vi "line_test.vi"   [LabVIEW 2012]
uses:
  <vilib>/NXT/Dual Mode Library/Display/drawLine.vi
  <vilib>/NXT/Dual Mode Library/Waits/Wait_Num.vi
types:
  T1 = cluster{"Start X":i16, "Start X":i16, "Start X":i16, "Start X":i16}
  T2 = typedef "LVHSConnector.ctl" = cluster{"Hardware":string, "Flattened String":string}
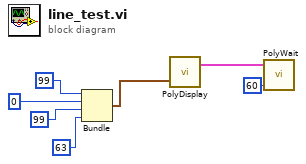
[diagram p0: block diagram]
diagram:
  n1 = Bundle("Start X"=i16 99, "Start X"=i16 0, "Start X"=i16 99, "Start X"=i16 63) -> (w4:T1)  [unwired: 1 in]
  n2 = call-poly <vilib>:"PolyDisplay.vi"("Line Parameters"=w4) -> ("NXT"=w6:T2)  [unwired: 3 in]
  n3 = call-poly <vilib>:"PolyWait.vi"("Time (1 sec)"=i16 60 ("Start X"), "NXT"=w6) -> ()  [unwired: 2 in, 1 out]
